vi "practica9a.vi"() -> ()   [LabVIEW 2013]
uses:
  <vilib>/measure/NI_MABase.lvlib
panel:
  out "Waveform Graph":waveform(dbl)(graph)
  in  "URL":string
  in  "stop":bool
  in  "signal type":T1(ring)
  in  "fase":dbl(knob) scale=0.0..10.0
  in  "amplitud":dbl(knob) scale=0.0..10.0
  in  "frecuencia":dbl(knob) scale=0.0..10.0
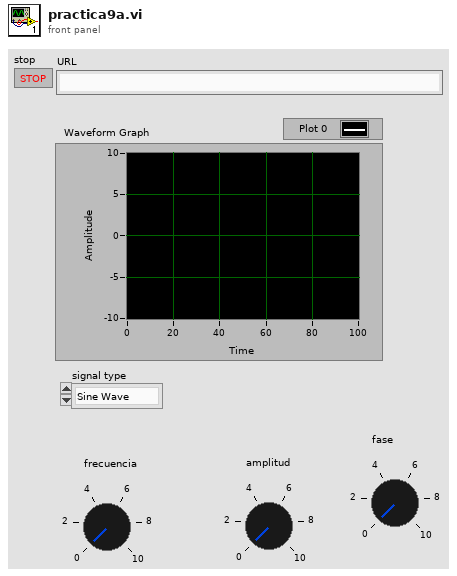
[diagram p1: front panel]
types:
  T1 = enum16{"Sine Wave", "Triangle Wave", "Square Wave", "Sawtooth Wave"}
  T2 = enum16{"Read", "Write", "ReadWrite", "BufferedRead", "BufferedReadWrite"}
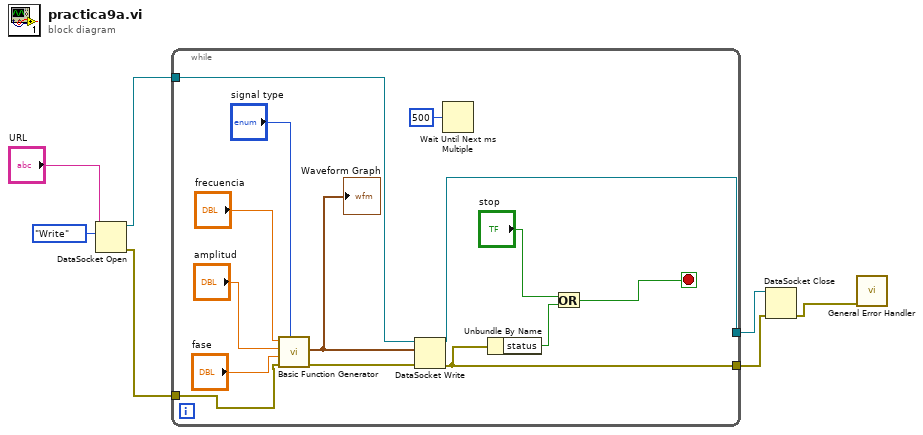
[diagram p0: block diagram]
diagram:
  n1 = DataSocket Open(10:T2."Write" ("mode"), 11:"URL") -> (0:w7:errorcluster, 3:w6:refnum<k13>)  [unwired: 2 in]
  n2 = while {
    tunnel: w7 -> [w17]
    tunnel: w6 -> [w15]
    tunnel: [w10] -> w5
    tunnel: [w9] -> w4
    stop <- w11 stop-if-true
    n3 = call <vilib>:"Basic Function Generator.vi"("signal type"="signal type", "error in (no error)"=w17, "phase"="fase", "amplitude"="amplitud", "frequency"="frecuencia") -> ("error out"=w16:errorcluster, "signal out"=w8:waveform(dbl))  [unwired: 4 in, 1 out]
    "Waveform Graph" <- w8
    n4 = DataSocket Write(8:w16, 10:w8, 11:w15) -> (0:w10:errorcluster, 3:w9:refnum<k13>)  [unwired: 1 in, 1 out]
    n5 = Wait Until Next ms Multiple(millisecond multiple=u32 500) -> ()  [unwired: 1 out]
    n6 = Unbundle By Name(w10) -> ("status"=w12:bool)
    n7 = Or(x="stop", y=w12) -> (x .or. y?=w11:bool)
  }
  n8 = DataSocket Close(8:w5, 11:w4) -> (0:w3:errorcluster)  [unwired: 1 in, 1 out]
  n9 = call <vilib>:"General Error Handler.vi"("error in (no error)"=w3) -> ()  [unwired: 10 in, 5 out]
